vi "TMCM351-Demo.vi"() -> ()   [LabVIEW 2018]
uses:
  <vilib>/Instr/_visa.llb/VISA Configure Serial Port (Instr).vi
panel:
  in  "停止":bool
  in  "Speed":i32=100 min=0 max=2047
  out "错误输出":errorcluster
  in  "Z归0":bool
  in  "Y 归0":bool
  in  "X 归0":bool
  out "当前位置":string[](array[string])
  in  "Z 连续反转":bool
  in  "Z 连续正转":bool
  in  "Y 连续反转":bool
  in  "Y 连续正转":bool
  in  "X 连续反转":bool
  in  "X 连续正转":bool
  in  "制动":bool
  out "Z Left":bool caption="Left"
  out "Z Right":bool caption="Right"
  out "Y Left":bool caption="Left"
  out "Y Right":bool caption="Right"
  out "X Lift":bool caption="Left"
  out "X Right":bool caption="Right"
  in  "Z 启动":bool
  in  "Y 启动":bool
  in  "X 启动":bool
  in  "Step Z":i32 min=-8388607 max=8388607
  in  "Step Y":i32 min=-8388607 max=8388607
  in  "Step X":i32 min=-8388607 max=8388607
  in  "Step COM":refnum<visa-resource-name>="COM5"
  # "X"
  # "Y"
  # "Z"
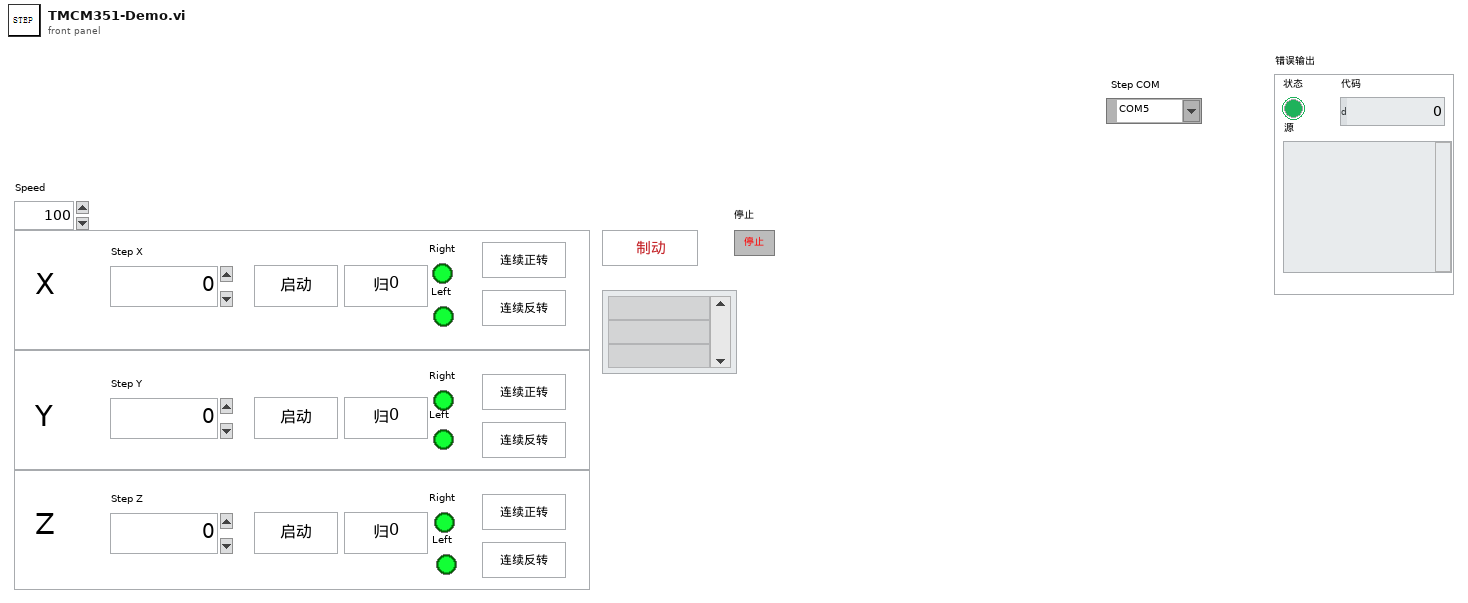
[diagram p1: front panel]
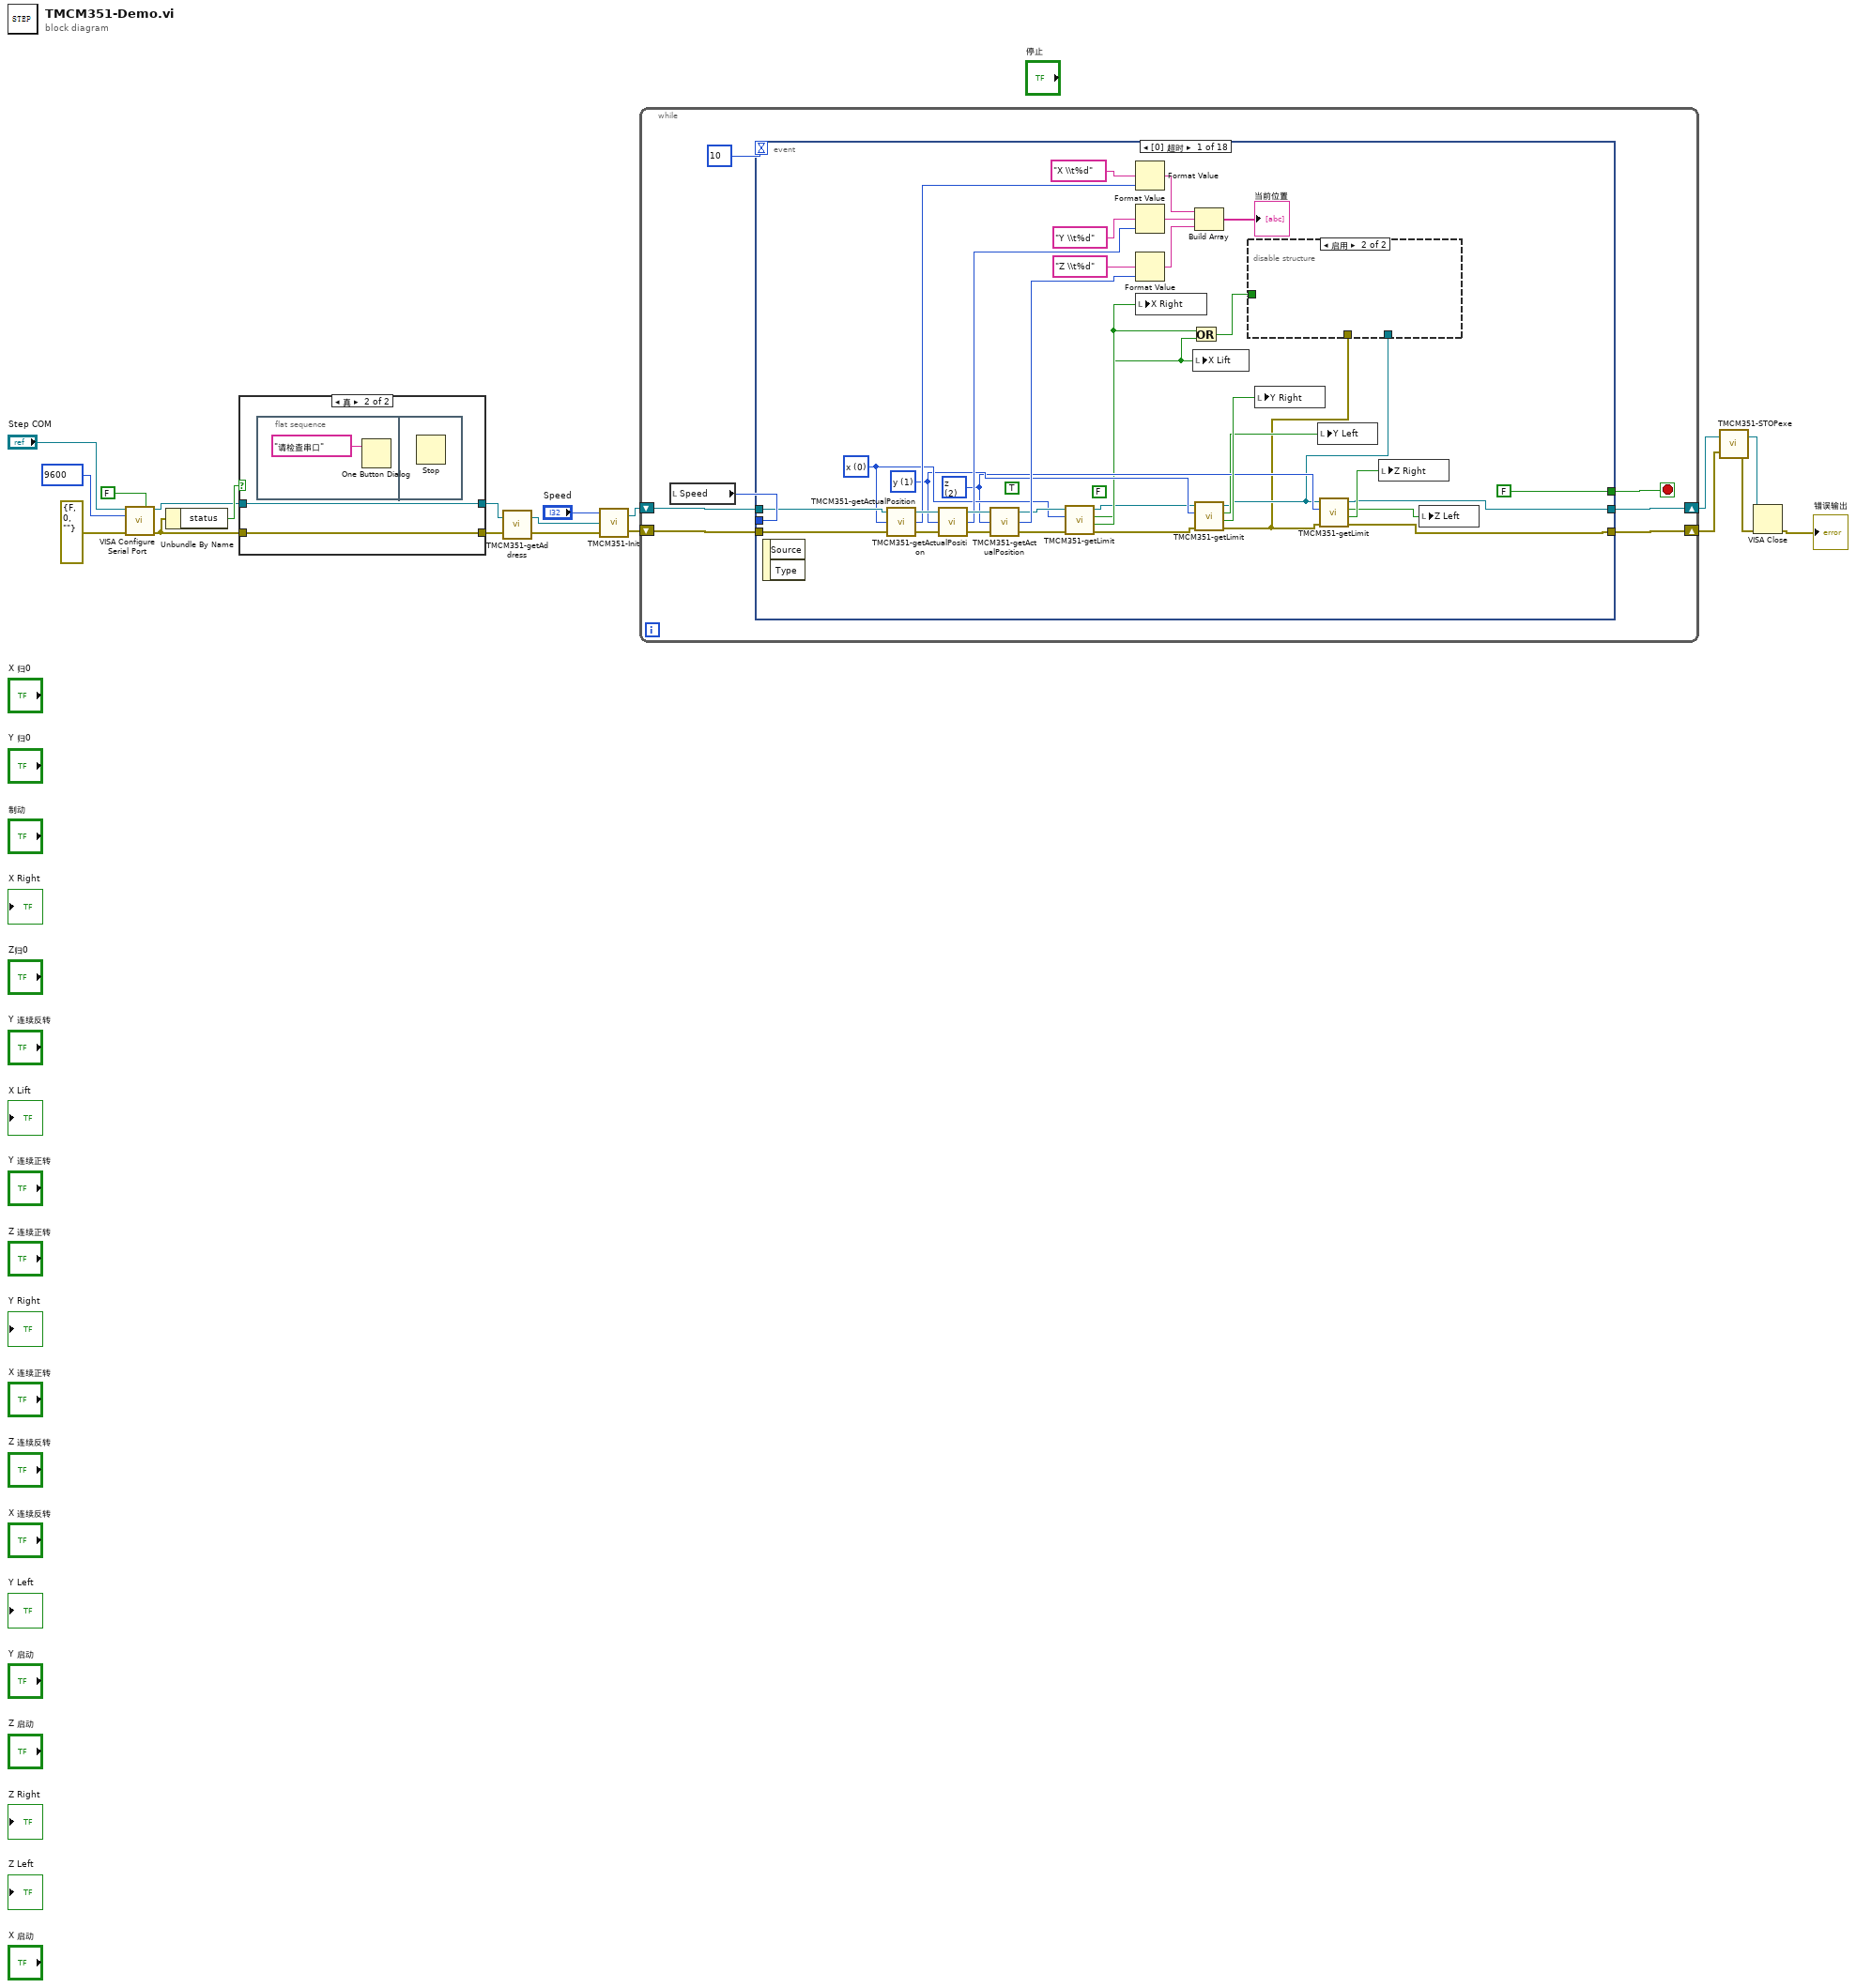
[diagram p0: block diagram]
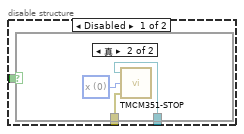
[diagram p3: hidden frame]
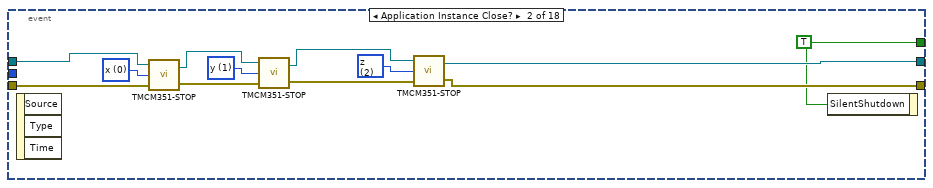
[diagram p5: hidden frame]
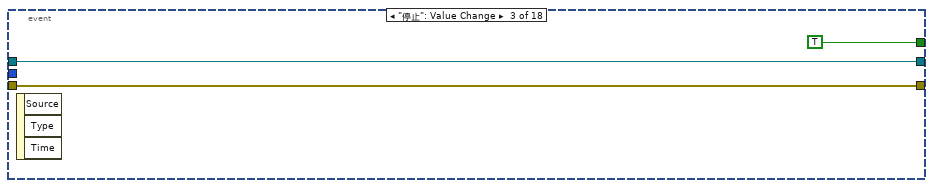
[diagram p6: hidden frame]
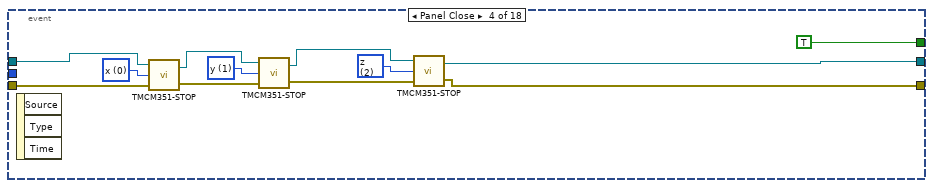
[diagram p7: hidden frame]
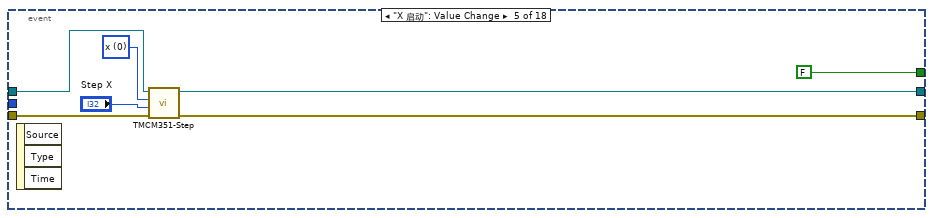
[diagram p8: hidden frame]
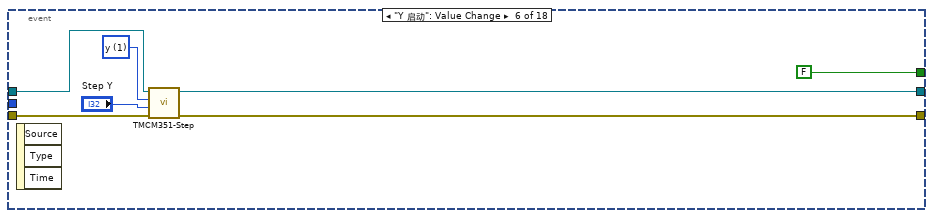
[diagram p9: hidden frame]
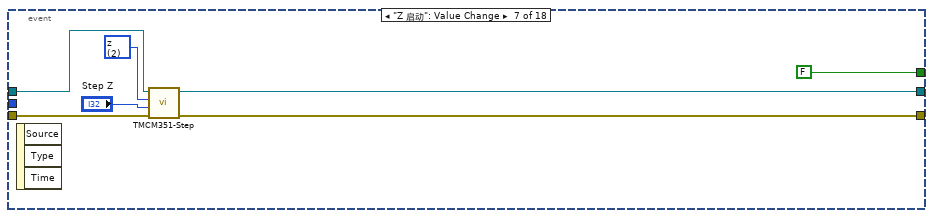
[diagram p10: hidden frame]
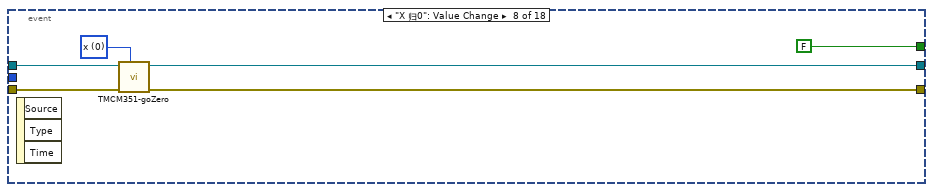
[diagram p11: hidden frame]
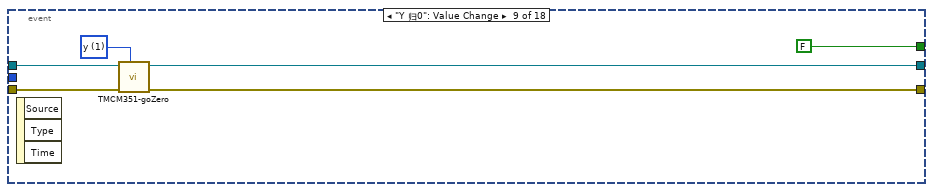
[diagram p12: hidden frame]
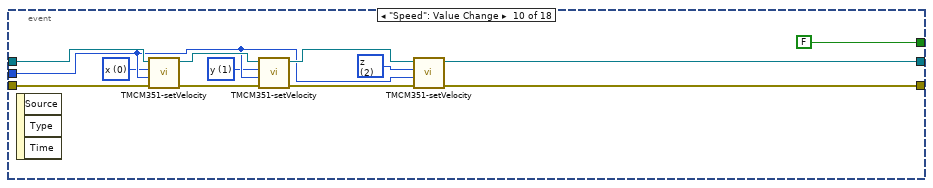
[diagram p13: hidden frame]
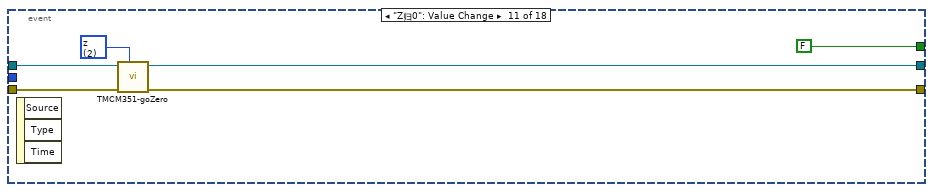
[diagram p14: hidden frame]
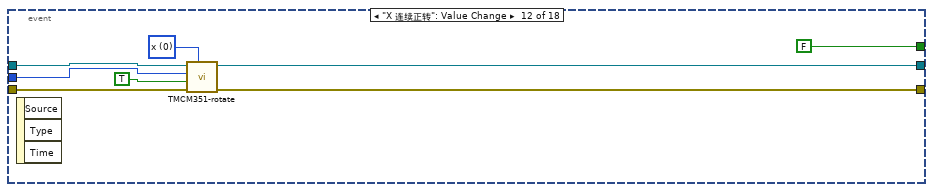
[diagram p15: hidden frame]
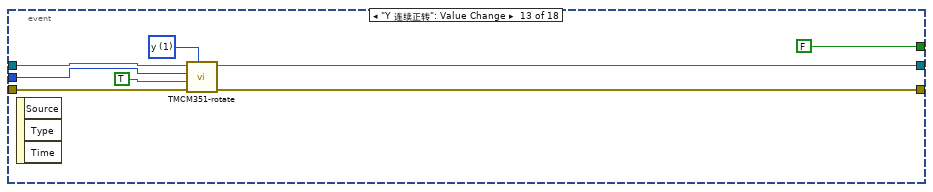
[diagram p16: hidden frame]
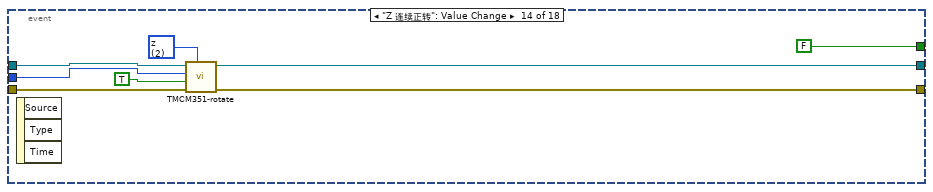
[diagram p17: hidden frame]
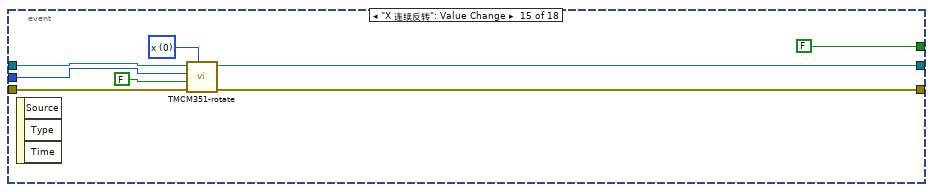
[diagram p18: hidden frame]
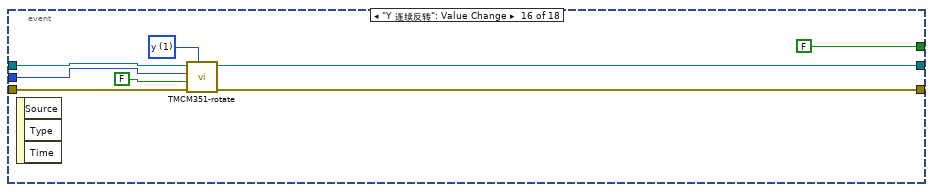
[diagram p19: hidden frame]
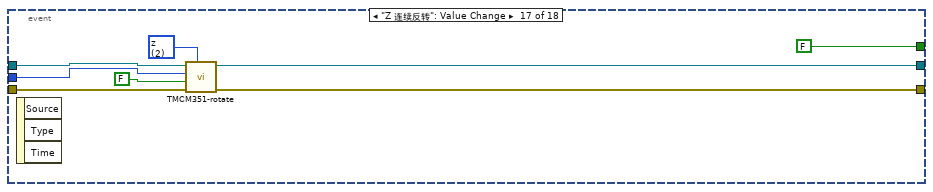
[diagram p20: hidden frame]
diagram:
  n1 = call-poly "VISA Configure Serial Port"("VISA resource name"="Step COM", "Enable Termination\nChar (T)"=FALSE ("Enable Termination\nChar (T)"), "baud rate (9600)"=u32 9600, "error in (no error)"=errorcluster {"status"=FALSE, "code"=0, "source"=""}) -> ("VISA resource name out"=w14:refnum<visa-resource-name>, "error out"=w13:errorcluster)  [unwired: 10 in]
  n2 = Unbundle By Name(w13) -> ("status"=w15:bool)
  n3 = case shown="真" w15 {
    tunnel: w14 -> [w21 w23]
    tunnel: w13 -> [w20 w22]
    tunnel: [w21 w23] -> w12
    tunnel: [w20 w22] -> w11
    frame False {
    }
    frame True {
      n4 = flat-sequence {
        frame #0 {
          n5 = One Button Dialog(message="请检查串口" ("消息")) -> ()  [unwired: 1 in, 1 out]
        }
        frame #1 {
          n6 = Stop() -> ()  [unwired: 1 in]
        }
      }
    }
  }
  n7 = call "TMCM351-getAddress.vi"("错误输入"=w11, "com in"=w12) -> ("错误输出"=w9:errorcluster, "com out"=w10:refnum<visa-resource-name>)
  n8 = call "TMCM351-Init.vi"("错误输入"=w9, "com in"=w10, "Speed"="Speed") -> ("错误输出"=w7:errorcluster, "com out"=w8:refnum<visa-resource-name>)
  n9 = while {
    shift-right: [w29] -> w3
    shift-left: w7 -> [w30]
    shift-right: [w28] -> w4
    shift-left: w8 -> [w27]
    stop <- w26 stop-if-true
    n10 = local read "Speed"() -> (w25:i32)
    n11 = event shown="[0] 超时" {
      selector: _ -> [_ _ _ _ _ _ _ _ _ _ _ _ _ _ _ _ _ _]
      dyn-events: _ -> [_ _ _ _ _ _ _ _ _ _ _ _ _ _ _ _ _ _]
      timeout: 10 -> [_ _ _ _ _ _ _ _ _ _ _ _ _ _ _ _ _ _]
      tunnel: w30 -> [w65 w76 w85 w90 w105 w111 w118 w124 w130 w140 w149 w153 w164 w169 w177 w185 w193 w209]
      tunnel: [w36 w74 w85 w88 w103 w109 w117 w122 w129 w134 w148 w152 w163 w168 w176 w184 w192 w200] -> w29
      tunnel: [w37 w75 w86 w89 w104 w110 w116 w123 w128 w135 w147 w157 w165 w172 w181 w189 w197 w201] -> w28
      tunnel: w27 -> [w61 w77 w86 w91 w106 w112 w119 w125 w131 w141 w150 w158 w166 w173 w182 w190 w198 w211]
      tunnel: [FALSE w73 TRUE TRUE FALSE FALSE FALSE FALSE FALSE FALSE FALSE FALSE FALSE FALSE FALSE FALSE FALSE FALSE] -> w26
      tunnel: w25 -> [_ _ _ _ _ _ _ _ _ w139 _ w155 w161 w171 w179 w187 w195 _]
      event Timeout {
        (unwired) FALSE
        (unwired) TRUE ("right?")
        w43 = u8 2 items=["x", "y", "z"] ("motor")
        w45 = u8 1 items=["x", "y", "z"] ("motor")
        w47 = u8 0 items=["x", "y", "z"] ("motor")
        n12 = event-data() -> ()  [unwired: 1 in, 2 out]
        n13 = call "TMCM351-getActualPosition.vi"("错误输入"=w65, "motor"=w47, "com in"=w61) -> ("错误输出"=w64:errorcluster, "Pisotion"=w52:i32, "com out"=w66:refnum<visa-resource-name>)
        n14 = call "TMCM351-getActualPosition.vi"("错误输入"=w64, "motor"=w45, "com in"=w66) -> ("错误输出"=w63:errorcluster, "Pisotion"=w51:i32, "com out"=w62:refnum<visa-resource-name>)
        n15 = call "TMCM351-getActualPosition.vi"("错误输入"=w63, "motor"=w43, "com in"=w62) -> ("错误输出"=w48:errorcluster, "Pisotion"=w50:i32, "com out"=w49:refnum<visa-resource-name>)
        n16 = call "TMCM351-getLimit.vi"("错误输入"=w48, "motor"=w47, "com in"=w49) -> ("错误输出"=w39:errorcluster, "right limit"=w42:bool, "left limit"=w34:bool, "com out"=w40:refnum<visa-resource-name>)  [unwired: 1 in]
        n17 = Format Value(format string="X \\t%d" ("格式字符串"), value (0)=w52) -> (output string=w57:string)  [unwired: 1 in]
        n18 = Format Value(format string="Y \\t%d" ("格式字符串"), value (0)=w51) -> (output string=w55:string)  [unwired: 1 in]
        n19 = Format Value(format string="Z \\t%d" ("格式字符串"), value (0)=w50) -> (output string=w53:string)  [unwired: 1 in]
        n20 = local write "X Right"(w42) -> ()
        n21 = Or(x=w42, y=w34) -> (x .or. y?=w41:bool)
        n22 = local write "X Lift"(w34) -> ()
        n23 = Build Array(w57, w55, w53) -> (→"当前位置":string[])
        n24 = call "TMCM351-getLimit.vi"("错误输入"=w39, "motor"=w45, "com in"=w40) -> ("错误输出"=w32:errorcluster, "right limit"=w46:bool, "left limit"=w38:bool, "com out"=w33:refnum<visa-resource-name>)  [unwired: 1 in]
        n25 = disable-structure shown="启用" {
          disable-tunnel: w41 -> [w69 _]
          disable-tunnel: w33 -> [w68 _]
          disable-tunnel: w32 -> [w67 _]
          frame Disabled {
            n26 = case shown="真" w69 {
              tunnel: w68 -> [_ w71]
              tunnel: w67 -> [_ w70]
              frame False {
              }
              frame True {
                w72 = u8 0 items=["x", "y", "z"] ("motor")
                n27 = call "TMCM351-STOP.vi"("错误输入"=w70, "motor"=w72, "com in"=w71) -> ()  [unwired: 2 out]
              }
            }
          }
          frame Enabled {
          }
        }
        n28 = local write "Y Right"(w46) -> ()
        n29 = local write "Y Left"(w38) -> ()
        n30 = call "TMCM351-getLimit.vi"("错误输入"=w32, "motor"=w43, "com in"=w33) -> ("错误输出"=w36:errorcluster, "right limit"=w44:bool, "left limit"=w35:bool, "com out"=w37:refnum<visa-resource-name>)  [unwired: 1 in]
        n31 = local write "Z Right"(w44) -> ()
        n32 = local write "Z Left"(w35) -> ()
      }
      event Application Instance Close? {
        w78 = u8 2 items=["x", "y", "z"] ("motor")
        w79 = u8 1 items=["x", "y", "z"] ("motor")
        w84 = u8 0 items=["x", "y", "z"] ("motor")
        w73 = TRUE
        n33 = event-data() -> ()  [unwired: 1 in, 3 out]
        n34 = call "TMCM351-STOP.vi"("错误输入"=w76, "motor"=w84, "com in"=w77) -> ("错误输出"=w83:errorcluster, "com out"=w82:refnum<visa-resource-name>)
        n35 = call "TMCM351-STOP.vi"("错误输入"=w83, "motor"=w79, "com in"=w82) -> ("错误输出"=w81:errorcluster, "com out"=w80:refnum<visa-resource-name>)
        n36 = call "TMCM351-STOP.vi"("错误输入"=w81, "motor"=w78, "com in"=w80) -> ("错误输出"=w74:errorcluster, "com out"=w75:refnum<visa-resource-name>)
        n37 = event-data("SilentShutdown"=w73) -> ()  [unwired: 1 in, 1 out]
      }
      event "停止": Value Change {
        n38 = event-data() -> ()  [unwired: 1 in, 3 out]
      }
      event Panel Close {
        w92 = u8 2 items=["x", "y", "z"] ("motor")
        w93 = u8 1 items=["x", "y", "z"] ("motor")
        w98 = u8 0 items=["x", "y", "z"] ("motor")
        n39 = event-data() -> ()  [unwired: 1 in, 3 out]
        n40 = call "TMCM351-STOP.vi"("错误输入"=w90, "motor"=w98, "com in"=w91) -> ("错误输出"=w97:errorcluster, "com out"=w96:refnum<visa-resource-name>)
        n41 = call "TMCM351-STOP.vi"("错误输入"=w97, "motor"=w93, "com in"=w96) -> ("错误输出"=w95:errorcluster, "com out"=w94:refnum<visa-resource-name>)
        n42 = call "TMCM351-STOP.vi"("错误输入"=w95, "motor"=w92, "com in"=w94) -> ("错误输出"=w88:errorcluster, "com out"=w89:refnum<visa-resource-name>)
      }
      event "X 启动": Value Change {
        w101 = u8 0 items=["x", "y", "z"] ("motor")
        n43 = event-data() -> ()  [unwired: 1 in, 3 out]
        n44 = call "TMCM351-Step.vi"("错误输入"=w105, "Step"="Step X", "motor"=w101, "com in"=w106) -> ("错误输出"=w103:errorcluster, "com out"=w104:refnum<visa-resource-name>)  [unwired: 2 in]
      }
      event "Y 启动": Value Change {
        w113 = u8 1 items=["x", "y", "z"] ("motor")
        n45 = event-data() -> ()  [unwired: 1 in, 3 out]
        n46 = call "TMCM351-Step.vi"("错误输入"=w111, "Step"="Step Y", "motor"=w113, "com in"=w112) -> ("错误输出"=w109:errorcluster, "com out"=w110:refnum<visa-resource-name>)  [unwired: 2 in]
      }
      event "Z 启动": Value Change {
        w120 = u8 2 items=["x", "y", "z"] ("motor")
        n47 = event-data() -> ()  [unwired: 1 in, 3 out]
        n48 = call "TMCM351-Step.vi"("错误输入"=w118, "Step"="Step Z", "motor"=w120, "com in"=w119) -> ("错误输出"=w117:errorcluster, "com out"=w116:refnum<visa-resource-name>)  [unwired: 2 in]
      }
      event "X 归0": Value Change {
        w121 = u8 0 items=["x", "y", "z"] ("motor")
        n49 = event-data() -> ()  [unwired: 1 in, 3 out]
        n50 = call "TMCM351-goZero.vi"("motor"=w121, "错误输入"=w124, "com in"=w125) -> ("错误输出"=w122:errorcluster, "com out"=w123:refnum<visa-resource-name>)  [unwired: 4 in]
      }
      event "Y 归0": Value Change {
        w132 = u8 1 items=["x", "y", "z"] ("motor")
        n51 = event-data() -> ()  [unwired: 1 in, 3 out]
        n52 = call "TMCM351-goZero.vi"("motor"=w132, "错误输入"=w130, "com in"=w131) -> ("错误输出"=w129:errorcluster, "com out"=w128:refnum<visa-resource-name>)  [unwired: 4 in]
      }
      event "Speed": Value Change {
        w136 = u8 2 items=["x", "y", "z"] ("motor")
        w137 = u8 1 items=["x", "y", "z"] ("motor")
        w138 = u8 0 items=["x", "y", "z"] ("motor")
        n53 = event-data() -> ()  [unwired: 1 in, 3 out]
        n54 = call "TMCM351-setVelocity.vi"("错误输入"=w140, "Speed"=w139, "motor"=w138, "com in"=w141) -> ("错误输出"=w145:errorcluster, "com out"=w144:refnum<visa-resource-name>)  [unwired: 2 in]
        n55 = call "TMCM351-setVelocity.vi"("错误输入"=w145, "Speed"=w139, "motor"=w137, "com in"=w144) -> ("错误输出"=w143:errorcluster, "com out"=w142:refnum<visa-resource-name>)  [unwired: 2 in]
        n56 = call "TMCM351-setVelocity.vi"("错误输入"=w143, "Speed"=w139, "motor"=w136, "com in"=w142) -> ("错误输出"=w134:errorcluster, "com out"=w135:refnum<visa-resource-name>)  [unwired: 2 in]
      }
      event "Z归0": Value Change {
        w151 = u8 2 items=["x", "y", "z"] ("motor")
        n57 = event-data() -> ()  [unwired: 1 in, 3 out]
        n58 = call "TMCM351-goZero.vi"("motor"=w151, "错误输入"=w149, "com in"=w150) -> ("错误输出"=w148:errorcluster, "com out"=w147:refnum<visa-resource-name>)  [unwired: 4 in]
      }
      event "X 连续正转": Value Change {
        w156 = u8 0 items=["x", "y", "z"] ("motor")
        n59 = event-data() -> ()  [unwired: 1 in, 3 out]
        n60 = call "TMCM351-rotate.vi"("motor"=w156, "错误输入"=w153, "正转？"=TRUE, "Speed"=w155, "com in"=w158) -> ("错误输出"=w152:errorcluster, "com out"=w157:refnum<visa-resource-name>)  [unwired: 2 in]
      }
      event "Y 连续正转": Value Change {
        w162 = u8 1 items=["x", "y", "z"] ("motor")
        n61 = event-data() -> ()  [unwired: 1 in, 3 out]
        n62 = call "TMCM351-rotate.vi"("motor"=w162, "错误输入"=w164, "正转？"=TRUE, "Speed"=w161, "com in"=w166) -> ("错误输出"=w163:errorcluster, "com out"=w165:refnum<visa-resource-name>)  [unwired: 2 in]
      }
      event "Z 连续正转": Value Change {
        w174 = u8 2 items=["x", "y", "z"] ("motor")
        n63 = event-data() -> ()  [unwired: 1 in, 3 out]
        n64 = call "TMCM351-rotate.vi"("motor"=w174, "错误输入"=w169, "正转？"=TRUE, "Speed"=w171, "com in"=w173) -> ("错误输出"=w168:errorcluster, "com out"=w172:refnum<visa-resource-name>)  [unwired: 2 in]
      }
      event "X 连续反转": Value Change {
        w180 = u8 0 items=["x", "y", "z"] ("motor")
        n65 = event-data() -> ()  [unwired: 1 in, 3 out]
        n66 = call "TMCM351-rotate.vi"("motor"=w180, "错误输入"=w177, "正转？"=FALSE, "Speed"=w179, "com in"=w182) -> ("错误输出"=w176:errorcluster, "com out"=w181:refnum<visa-resource-name>)  [unwired: 2 in]
      }
      event "Y 连续反转": Value Change {
        w188 = u8 1 items=["x", "y", "z"] ("motor")
        n67 = event-data() -> ()  [unwired: 1 in, 3 out]
        n68 = call "TMCM351-rotate.vi"("motor"=w188, "错误输入"=w185, "正转？"=FALSE, "Speed"=w187, "com in"=w190) -> ("错误输出"=w184:errorcluster, "com out"=w189:refnum<visa-resource-name>)  [unwired: 2 in]
      }
      event "Z 连续反转": Value Change {
        w196 = u8 2 items=["x", "y", "z"] ("motor")
        n69 = event-data() -> ()  [unwired: 1 in, 3 out]
        n70 = call "TMCM351-rotate.vi"("motor"=w196, "错误输入"=w193, "正转？"=FALSE, "Speed"=w195, "com in"=w198) -> ("错误输出"=w192:errorcluster, "com out"=w197:refnum<visa-resource-name>)  [unwired: 2 in]
      }
      event "制动": Value Change {
        w202 = u8 2 items=["x", "y", "z"] ("motor")
        w203 = u8 1 items=["x", "y", "z"] ("motor")
        w208 = u8 0 items=["x", "y", "z"] ("motor")
        n71 = event-data() -> ()  [unwired: 1 in, 3 out]
        n72 = call "TMCM351-STOP.vi"("错误输入"=w209, "motor"=w208, "com in"=w211) -> ("错误输出"=w207:errorcluster, "com out"=w206:refnum<visa-resource-name>)
        n73 = call "TMCM351-STOP.vi"("错误输入"=w207, "motor"=w203, "com in"=w206) -> ("错误输出"=w205:errorcluster, "com out"=w204:refnum<visa-resource-name>)
        n74 = call "TMCM351-STOP.vi"("错误输入"=w205, "motor"=w202, "com in"=w204) -> ("错误输出"=w200:errorcluster, "com out"=w201:refnum<visa-resource-name>)
      }
    }
  }
  n75 = call "TMCM351-STOPexe.vi"("错误输入"=w3, "com in"=w4) -> ("错误输出"=w1:errorcluster, "com out"=w2:refnum<visa-resource-name>)
  n76 = VISA Close(VISA resource name=w2, error in (no error)=w1) -> (error out=→"错误输出":errorcluster)
